vi "SaveExperimentDataToAsciiFile.vi"(8 "error in (no error)":errorcluster, 11 "Ascii Experiment Data":T1) -> (0 "error out":errorcluster)   [LabVIEW 2013]
doc: "Use this template to build a VI to use as a subVI."
uses:
  Ascii Experiment Data.ctl
  DateandTime.ctl
  <vilib>/Utility/file.llb/Write To Spreadsheet File (string).vi
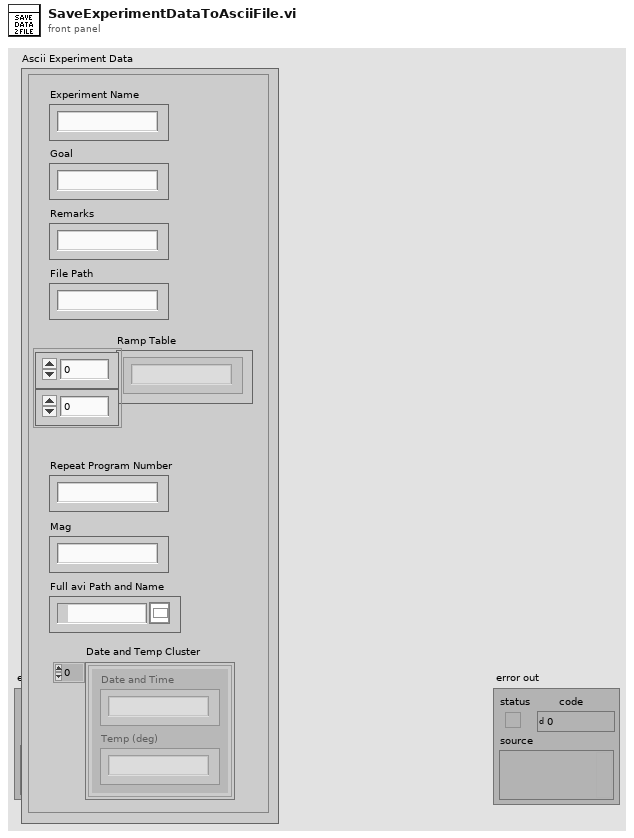
[diagram p1: front panel]
types:
  T1 = typedef "Ascii Experiment Data.ctl" = cluster{"Experiment Name":string, "Goal":string, "Remarks":string, "File Path":string, "Mag":string, "Repeat Program Number":string, "Full avi Path and Name":path, "Ramp Table ":string[][], "Date and Time":T2}
  T2 = typedef "DateandTime.ctl" = cluster{"Date and Time":string, "Temp (deg)":string}[]
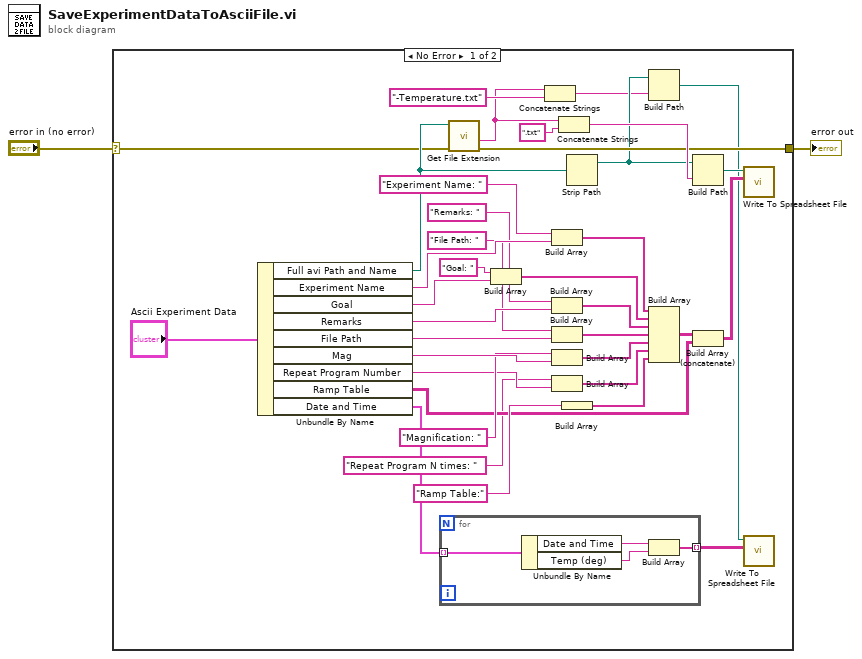
[diagram p0: block diagram]
diagram:
  n1 = case shown="No Error" "error in (no error)" {
    selector: "error in (no error)" -> [w37 w44]
    tunnel: [w34 w44] -> w1
    frame No Error {
      n2 = Unbundle By Name("Ascii Experiment Data") -> ("Full avi Path and Name"=w38:path, "Experiment Name"=w32:string, "Goal"=w27:string, "Remarks"=w24:string, "File Path"=w21:string, "Mag"=w18:string, "Repeat Program Number"=w12:string, "Ramp Table"=w13:string[][], "Date and Time"=w4:T2)
      n3 = for {
        tunnel: w4 -> [w43] mode=indexing
        tunnel: [w40] -> w3 mode=indexing
        n4 = Unbundle By Name(w43) -> ("Date and Time"=w42:string, "Temp (deg)"=w41:string)
        n5 = Build Array(w42, w41) -> (w40:string[])
      }
      n6 = call <vilib>:"Get File Extension.vi"("error in (no error)"=w37, "file"=w38) -> ("error out"=w34:errorcluster, "filename without extension"=w6:string)  [unwired: 6 in, 2 out]
      n7 = Build Array("Goal: " ("element"), w27) -> (w25:string[])
      n8 = Concatenate Strings(w6, "-Temperature.txt" ("string")) -> (w7:string)
      n9 = Build Array("Experiment Name: " ("element"), w32) -> (w30:string[])
      n10 = Build Array("Remarks: " ("element"), w24) -> (w22:string[])
      n11 = Build Array("File Path: " ("element"), w21) -> (w19:string[])
      n12 = Build Array("Magnification: " ("element"), w18) -> (w16:string[])
      n13 = Build Array("Repeat Program N times: " ("element"), w12) -> (w10:string[])
      n14 = Concatenate Strings(w6, ".txt" ("string")) -> (w35:string)
      n15 = Build Array("Ramp Table:" ("element")) -> (w14:string[])
      n16 = Strip Path(path=w38) -> (stripped path=w9:path)  [unwired: 1 out]
      n17 = Build Path(base path=w9, name or relative path=w7) -> (appended path=w5:path)
      n18 = Build Array(w30, w25, w22, w19, w16, w10, w14) -> (w29:string[][])
      n19 = Build Path(base path=w9, name or relative path=w35) -> (appended path=w33:path)
      n20 = Build Array (concatenate)(w29, w13) -> (w28:string[][])
      n21 = call-poly <vilib>:"Write To Spreadsheet File.vi"("2D data"=w28, "file path (dialog if empty)"=w33) -> ()  [unwired: 6 in, 1 out]
      n22 = call-poly <vilib>:"Write To Spreadsheet File.vi"("2D data"=w3, "file path (dialog if empty)"=w5) -> ()  [unwired: 6 in, 1 out]
    }
    frame Error {
    }
  }
  "error out" <- w1
